vi "Get_Styles.vi"   [LabVIEW 2025]
types:
  T1 = typedef "LVStringsAndValuesArrayTypeDef.ctl" = cluster{"String":string, "Value":ext}[]
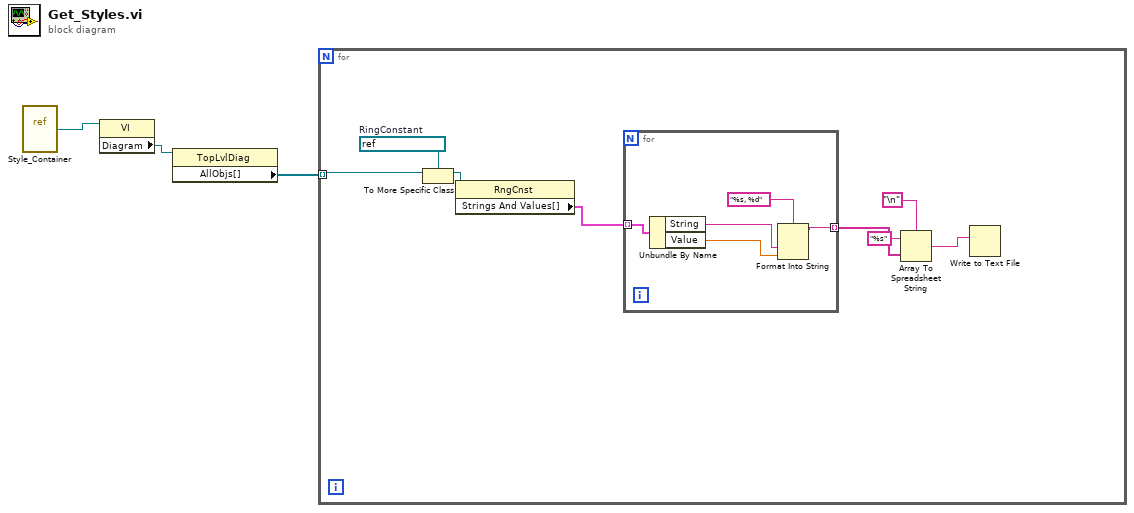
[diagram p0: block diagram]
diagram:
  n1 = vi-ref "Style_Container.vi"() -> (w3:refnum<vi>)
  n2 = property class="VI"(reference=w3) -> ("Diagram"=w2:refnum<vi>)  [unwired: 1 in, 2 out]
  n3 = property class="TopLvlDiag"(reference=w2) -> ("AllObjs[]"=w1:refnum<vi>[])  [unwired: 1 in, 2 out]
  n4 = for {
    tunnel: w1 -> [w11] mode=indexing
    w10 = refnum<vi> refnum  # RingConstant
    n5 = To More Specific Class(target class=w10, reference=w11) -> (specific class reference=w9:refnum<vi>)  [unwired: 1 in, 1 out]
    n6 = property class="RngCnst"(reference=w9) -> ("Strings And Values[]"=w8:T1)  [unwired: 1 in, 2 out]
    n7 = for {
      tunnel: w8 -> [w16] mode=indexing
      tunnel: [w12] -> w7 mode=indexing
      n8 = Unbundle By Name(w16) -> ("String"=w14:string, "Value"=w13:ext)
      n9 = Format Into String(format string="%s, %d", w14, w13) -> (resulting string=w12:string)  [unwired: 2 in, 1 out]
    }
    n10 = Array To Spreadsheet String(delimiter (Tab)="\n", array=w7, 3:"%s" ("format string")) -> (spreadsheet string=w4:string)
    n11 = Write to Text File(text=w4) -> ()  [unwired: 3 in, 3 out]
  }
